vi "CVT Add.vi"(7 "Group":string, 8 "error in":errorcluster, 9 "Data":variant, 10 "tag":string, 11 "cvt":refnum<data-value>) -> (0 "error out":errorcluster, 3 "cvt":refnum<data-value>)   [LabVIEW 2014]
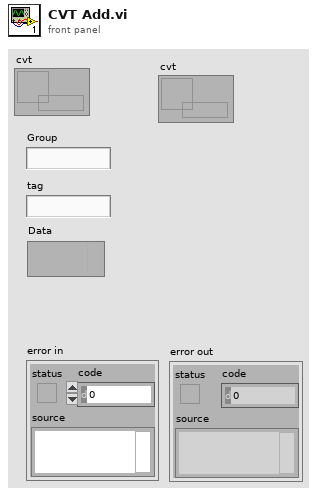
[diagram p1: front panel]
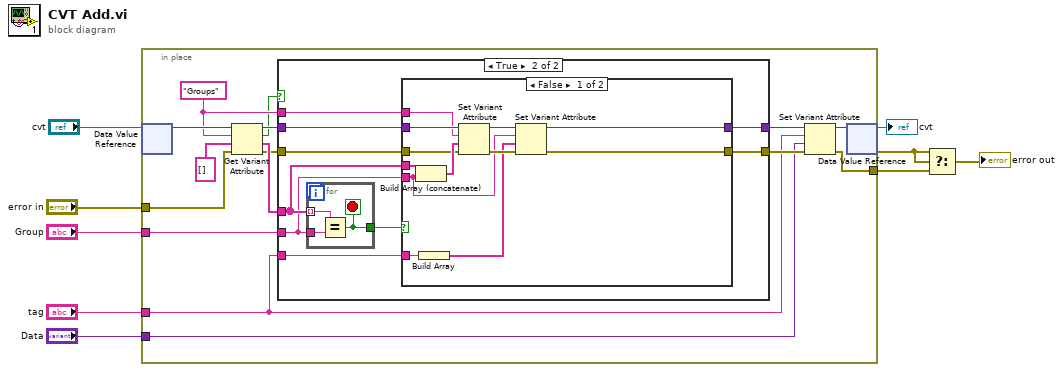
[diagram p0: block diagram]
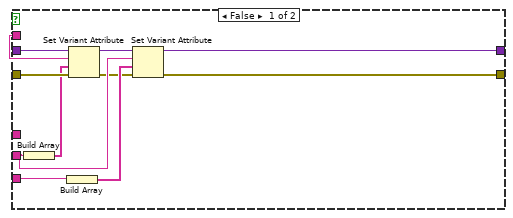
[diagram p2: hidden frame]
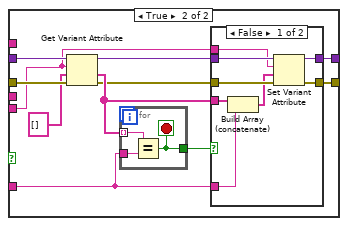
[diagram p3: hidden frame]
diagram:
  n1 = in-place {
    in-place-border: "Group" -> [w21]
    in-place-border: "tag" -> [w11]
    in-place-border: "Data" -> [w15]
    in-place-border: "error in" -> [w13]
    in-place-border: [w10] -> w4
    w20 = "Groups" ("name")
    n2 = in-place-dvr #1("cvt") -> (w24:variant)  [unwired: 1 out]
    n3 = Get Variant Attribute(Variant=w24, name=w20, default value (empty Variant)=string[] [], error in=w13) -> (duplicate Variant=w23:variant, found=w12:bool, value=w22:string[], error out=w19:errorcluster)
    n4 = case shown="True" w12 {
      tunnel: w23 -> [w35 w43]
      tunnel: w22 -> [_ w42]
      tunnel: w21 -> [w29 w41]
      tunnel: w20 -> [w33 w40]
      tunnel: w19 -> [w34 w39]
      tunnel: [w30 w37] -> w18
      tunnel: [w26 w36] -> w17
      tunnel: w11 -> [w28 w38]
      frame False {
        n5 = Build Array(w29) -> (w32:string[])
        n6 = Build Array(w28) -> (w27:string[])
        n7 = Set Variant Attribute(Variant=w35, name=w33, value=w32, error in=w34) -> (Variant out=w31:variant, error out=w25:errorcluster)  [unwired: 1 out]
        n8 = Set Variant Attribute(Variant=w31, name=w29, value=w27, error in=w25) -> (Variant out=w30:variant, error out=w26:errorcluster)  [unwired: 1 out]
      }
      frame True {
        n9 = for {
          tunnel: w42 -> [w82] mode=indexing
          tunnel: w41 -> [w83]
          tunnel: [w81] -> w44
          stop <- w81 stop-if-true
          n10 = Equal?(x=w82, y=w83) -> (x = y?=w81:bool)
        }
        n11 = case shown="False" w44 {
          tunnel: w43 -> [w56 w67]
          tunnel: w42 -> [w55 _]
          tunnel: w41 -> [w49 w57]
          tunnel: w40 -> [w53 _]
          tunnel: [w46 w58] -> w37
          tunnel: [w45 w59] -> w36
          tunnel: w39 -> [w52 w66]
          tunnel: w38 -> [w48 w61]
          frame False {
            n12 = Build Array (concatenate)(w55, w49) -> (w54:string[])
            n13 = Build Array(w48) -> (w47:string[])
            n14 = Set Variant Attribute(Variant=w56, name=w53, value=w54, error in=w52) -> (Variant out=w51:variant, error out=w50:errorcluster)  [unwired: 1 out]
            n15 = Set Variant Attribute(Variant=w51, name=w49, value=w47, error in=w50) -> (Variant out=w46:variant, error out=w45:errorcluster)  [unwired: 1 out]
          }
          frame True {
            n16 = Get Variant Attribute(Variant=w67, name=w57, default value (empty Variant)=string[] [], error in=w66) -> (duplicate Variant=w63:variant, value=w62:string[], error out=w60:errorcluster)  [unwired: 1 out]
            n17 = for {
              tunnel: w62 -> [w79] mode=indexing
              tunnel: w61 -> [w80]
              tunnel: [w78] -> w64
              stop <- w78 stop-if-true
              n18 = Equal?(x=w79, y=w80) -> (x = y?=w78:bool)
            }
            n19 = case shown="False" w64 {
              tunnel: w63 -> [w75 w77]
              tunnel: w62 -> [w74 _]
              tunnel: w61 -> [w73 _]
              tunnel: w60 -> [w72 w76]
              tunnel: [w71 w76] -> w59
              tunnel: [w70 w77] -> w58
              tunnel: w57 -> [w68 _]
              frame False {
                n20 = Build Array (concatenate)(w74, w73) -> (w69:string[])
                n21 = Set Variant Attribute(Variant=w75, name=w68, value=w69, error in=w72) -> (Variant out=w70:variant, error out=w71:errorcluster)  [unwired: 1 out]
              }
              frame True {
              }
            }
          }
        }
      }
    }
    n22 = Set Variant Attribute(Variant=w18, name=w11, value=w15, error in=w17) -> (Variant out=w14:variant, error out=w10:errorcluster)  [unwired: 1 out]
    n23 = in-place-dvr #1(w14) -> (→"cvt":refnum<data-value>, w5:errorcluster)
  }
  n24 = Select(t=w5, s=w5, f=w4) -> (s? t:f=→"error out":errorcluster)
